vi "Timing_LoopTime.vi"(3 "Loop Time In":u32) -> (0 "Runtime / s":dbl, 1 "Loop Time Out":u32)   [LabVIEW 2023]
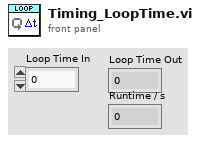
[diagram p1: front panel]
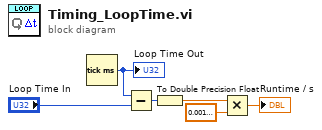
[diagram p0: block diagram]
diagram:
  n1 = Tick Count (ms)() -> (millisecond timer value=w6:u32)
  "Loop Time Out" <- w6
  n2 = Subtract(x=w6, y="Loop Time In") -> (x-y=w3:u32)
  n3 = To Double Precision Float(number=w3) -> (double precision float=w5:dbl)
  n4 = Multiply(x=w5, y=0.0010000000474974513) -> (x*y=→"Runtime / s":dbl)
